vi "Read Numeric Type.vi"(8 "error in (no error)":errorcluster, 11 "Number Writer in":refnum<class "Number Writer.lvclass">) -> (0 "error out":errorcluster, 2 "Numeric Type":T1=enum."I32", 3 "Number Writer out":refnum<class "Number Writer.lvclass">)   [LabVIEW 2013, in "Number Writer.lvclass"]
uses:
  Number Writer.lvclass
  Numeric Type.ctl
  Number Writer.lvclass/Number Writer.ctl
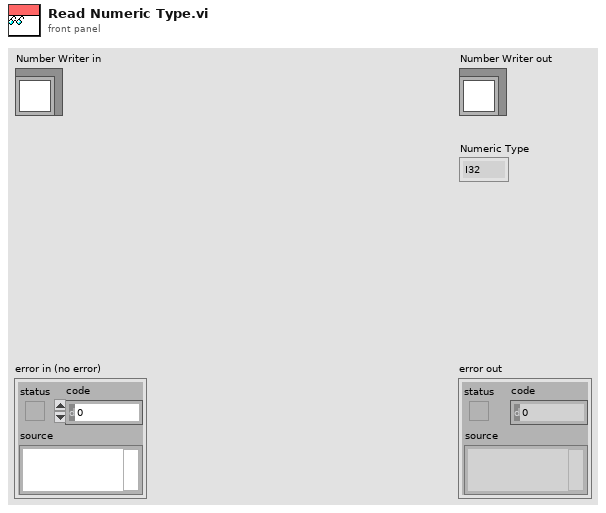
[diagram p1: front panel]
types:
  T1 = typedef "Number Writer.lvclass/Numeric Type.ctl" = enum16{"I8", "I16", "I32", "I64", "U8", "U16", "U32", "U64", "SGL", "DBL", "PTR INT", "PTR UINT"}
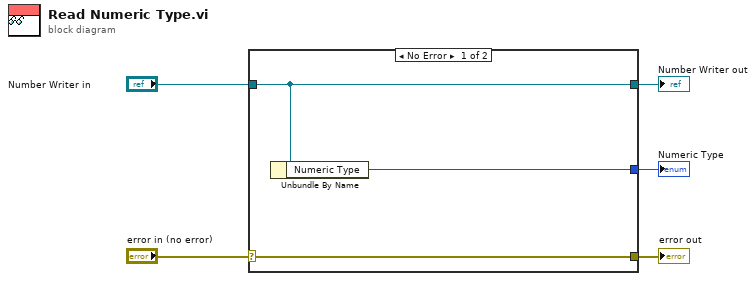
[diagram p0: block diagram]
diagram:
  n1 = case shown="No Error" "error in (no error)" {
    selector: "error in (no error)" -> [w8 w9]
    tunnel: [w8 w9] -> w4
    tunnel: [w7 w10] -> w2
    tunnel: "Number Writer in" -> [w7 w10]
    tunnel: [w6 _] -> w1
    frame No Error {
      n2 = Unbundle By Name(w7) -> ("Numeric Type"=w6:T1)
    }
    frame Error {
    }
  }
  "error out" <- w4
  "Number Writer out" <- w2
  "Numeric Type" <- w1
